vi "Hexadecimal to Octal.vi"(11 "Hexadecimal Number":i64 format="%x") -> (3 "Octal Number":i64 format="%o")   [LabVIEW 2020]
doc: "This VI will convert Hexadecimal Values to Octal Values."
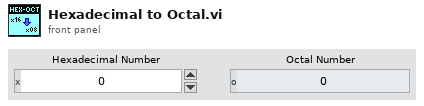
[diagram p1: front panel]
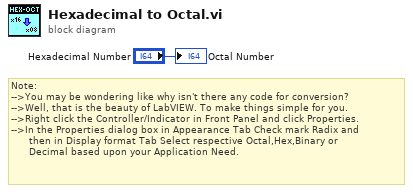
[diagram p0: block diagram]
diagram:
  # "Note: \n-->You may be wondering like why isn't there any code for conversion?\n-->Well, that is the beauty of LabVIEW. To make things simple for you.\n-->Right click the Controller/Indicator in Front Panel and click Properties.\n-->In the Properties dialog box in Appearance Tab Check mark Radix and \n      then in Display format Tab Select respective Octal,Hex,Binary or\n      Decimal based upon your Application Need."
  "Octal Number" <- "Hexadecimal Number"
